vi "PicoScope5000aSetupStreaming.vi"(0 "error in":errorcluster, 1 "Device Info":T2, 2 "handle in":i16, 3 "Acquisition Settings":T3={"Auto Stop"=FALSE, "Desired Sample Interval"=4, "Pre-trigger Samples"=0, "Post-trigger Samples"=1000, "Down-Sample Ratio"=1, "Down-Sample Mode"=0, "Time Units"=2} {"Time Units" items=["Nanoseconds (ns)"=2, "Microseconds (us)"=3, "Milliseconds (ms)"=4, "Seconds (s)"=5]; "Down-Sample Mode" items=["None"=0, "Aggregate"=1, "Decimate"=2, "Average"=4]}, 4 "Buffer and Transfer Settings":T1={"startIndex"=0, "Samples"=1000000, "Down Sample Ratio"=1, "Down-Sample Mode"=0} {"Down-Sample Mode" items=["None"=0, "Aggregate"=1, "Decimate"=2, "Average"=4]; "Down Sample Ratio" step=1; "Samples" format="%_6p"}, 5 "enabled array":i16[](array[numeric]), 10 "Pointers In":u64[][](array[numeric])) -> (11 "Pointer array":u64[][](array[numeric]), 14 "error out":errorcluster, 16 "handle out":i16, 17 "Sample Interval":u32, 19 "sampleIntervalTimeUnits":u32)   [LabVIEW 2016]
doc: "Set up the data buffers and calls RunStreaming to start the device streaming.\nData will be copied from the driver buffers into the corresponding application buffers using the wrapper dll."
uses:
  ps5000a.dll
  ps5000aWrap.dll
panel:
  # "Overview Buffer Size is the size of the temporary buffers used to\nstore data before returning it to the application."
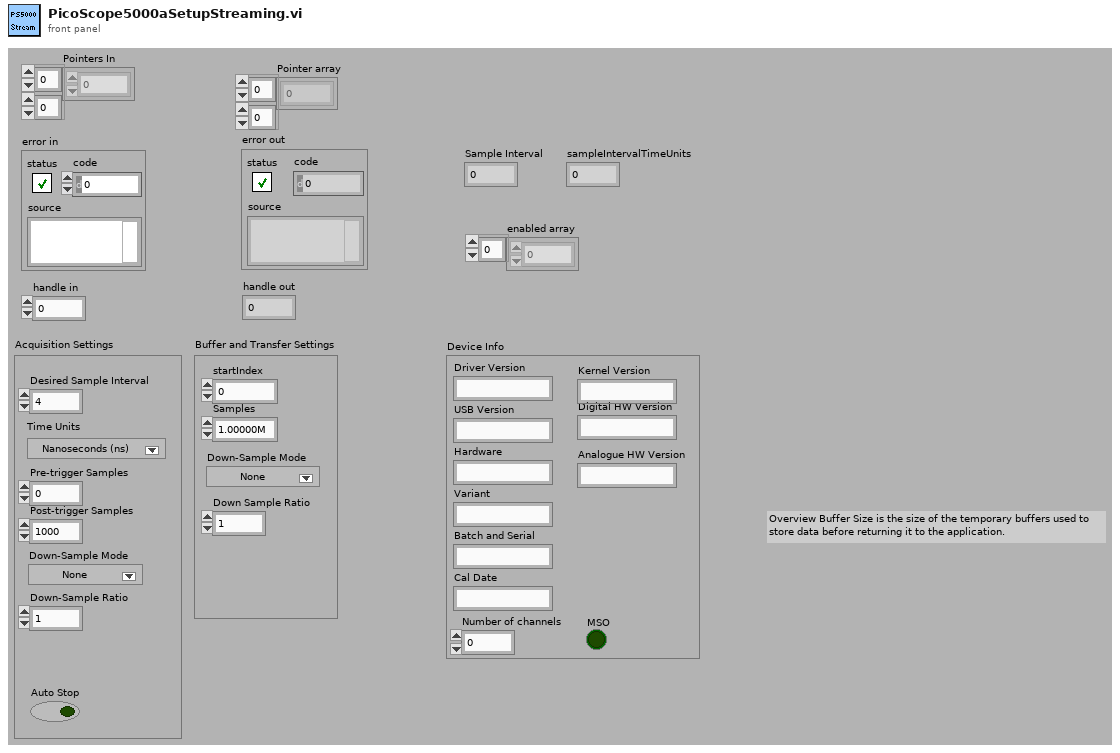
[diagram p1: front panel]
types:
  T1 = cluster{"startIndex":u64, "Samples":u64, "Down Sample Ratio":u64, "Down-Sample Mode":u32}
  T2 = cluster{"Driver Version":string, "USB Version":string, "Hardware":string, "Variant":string, "Batch and Serial":string, "Cal Date":string, "Kernel Version":string, "Digital HW Version":string, "Analogue HW Version":string, "MSO":bool, "Number of channels":i16}
  T3 = cluster{"Auto Stop":bool, "Desired Sample Interval":u32, "Pre-trigger Samples":u32, "Post-trigger Samples":u32, "Down-Sample Ratio":u32, "Down-Sample Mode":i32, "Time Units":u32}
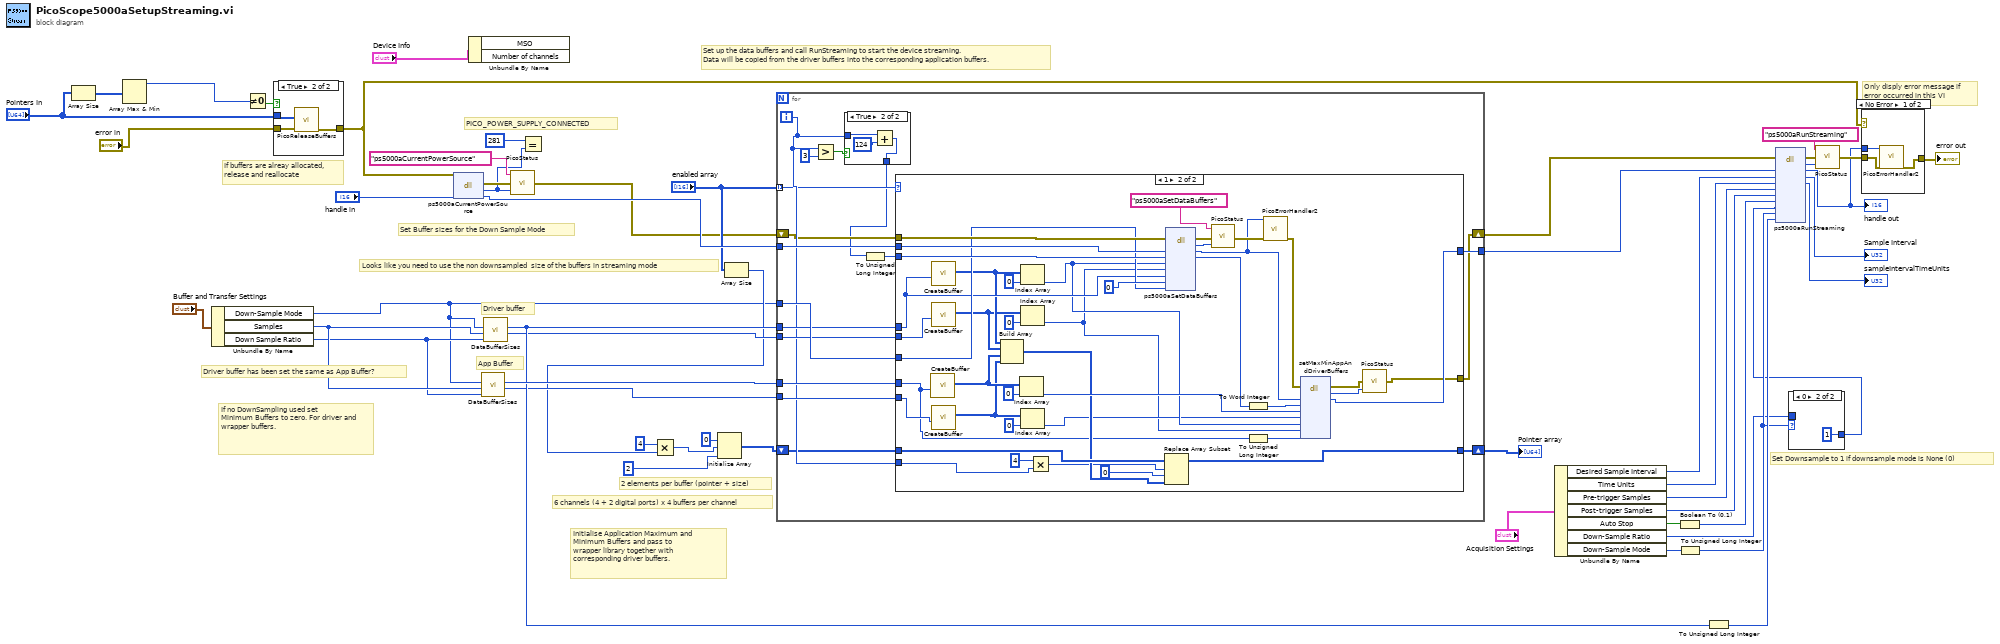
[diagram p0: block diagram]
diagram:
  # "Set Downsample to 1 if downsample mode is None (0)"
  # "Looks like you need to use the non downsampled  size of the buffers in streaming mode"
  # "If buffers are alreay allocated,\nrelease and reallocate"
  # "2 elements per buffer (pointer + size)"
  # "6 channels (4 + 2 digital ports) x 4 buffers per channel"
  # "App Buffer"
  # "Driver buffer"
  # "Driver buffer has been set the same as App Buffer?"
  # "Set Buffer sizes for the Down Sample Mode"
  # "If no DownSampling used set \nMinimum Buffers to zero. For driver and wrapper buffers."
  # "PICO_POWER_SUPPLY_CONNECTED"
  # "Initialise Application Maximum and\nMinimum Buffers and pass to \nwrapper library together with corresponding driver buffers."
  # "Only disply error message if\nerror occurred in this VI"
  # "Set up the data buffers and call RunStreaming to start the device streaming.\nData will be copied from the driver buffers into the corresponding application buffers."
  n1 = Array Size(array="Pointers In") -> (size(s)=w7:i32[])
  n2 = Array Max & Min(array=w7) -> (max value=w6:i32)  [unwired: 3 out]
  n3 = Unbundle By Name("Buffer and Transfer Settings") -> ("Down-Sample Mode"=w4:u32, "Samples"=w30:u64, "Down Sample Ratio"=w29:u64)
  n4 = Not Equal To 0?(x=w6) -> (x != 0?=w14:bool)
  n5 = case shown="True" w14 {
    tunnel: "Pointers In" -> [_ w54]
    tunnel: "error in" -> [w53 w55]
    tunnel: [w53 w56] -> w11
    frame False {
    }
    frame True {
      n6 = call "PicoReleaseBuffers.vi"("error in (no error)"=w55, "Pointer array"=w54) -> ("error out"=w56:errorcluster)  [unwired: 9 in]
    }
  }
  n7 = dll-call lib="ps5000a.dll" fn="ps5000aCurrentPowerSource"(error in=w11, "handle"="handle in") -> (error out=w37:errorcluster, "PICO_STATUS"=w35:u32, "handle"=w33:i16)  [unwired: 2 in, 1 out]
  n8 = Unbundle By Name("Device Info") -> ()  [unwired: 2 out]
  n9 = call "DataBufferSizes.vi"("Down Sample Ratio"=w29, "Number of Samples"=w30, "Down-Sample Mode"=w4) -> ("min Buffer Size"=w25:i32, "Max Buffer Size"=w28:i32)  [unwired: 7 in]
  n10 = call "DataBufferSizes.vi"("Down Sample Ratio"=w29, "Number of Samples"=w30, "Down-Sample Mode"=w4) -> ("min Buffer Size"=w26:i32, "Max Buffer Size"=w27:i32)  [unwired: 7 in]
  n11 = call "PicoStatus.vi"("PICO STATUS"=w35, "error in"=w37, "source"="ps5000aCurrentPowerSource") -> ("error out"=w10:errorcluster)
  n12 = Equal?(x=u32 281, y=w35) -> ()  [unwired: 1 out]
  n13 = Array Size(array="enabled array") -> (size(s)=w18:i32)
  n14 = Multiply(x=4, y=w18) -> (x*y=w19:i32)
  n15 = Initialize Array(u64 0 ("element"), w19, 2 ("dimension size")) -> (w8:u64[][])
  n16 = for {
    tunnel: "enabled array" -> [w62] mode=indexing
    tunnel: w33 -> [w73]
    tunnel: w4 -> [w72]
    tunnel: w28 -> [w71]
    tunnel: w27 -> [w70]
    tunnel: w26 -> [w69]
    tunnel: w25 -> [w68]
    tunnel: [w63] -> w21
    shift-right: [w61] -> w15
    shift-left: w10 -> [w60]
    shift-right: [w67] -> w24
    shift-left: w8 -> [w59]
    i -> [w64]
    n17 = Greater?(x=w64, y=3) -> (0:w65:bool)
    n18 = case shown="True" w65 {
      tunnel: [w74 w75] -> w57
      tunnel: w64 -> [w74 w77]
      frame False {
      }
      frame True {
        n19 = Add(x=w77, y=124) -> (x+y=w75:i32)
      }
    }
    n20 = To Unsigned Long Integer(number=w57) -> (unsigned 32bit integer=w58:u32)
    n21 = case shown="1" w62 {
      tunnel: w73 -> [w79 w121]
      tunnel: w60 -> [w78 w120]
      tunnel: w58 -> [_ w113]
      tunnel: w71 -> [_ w83]
      tunnel: w70 -> [_ w103]
      tunnel: w69 -> [_ w106]
      tunnel: w68 -> [_ w105]
      tunnel: w72 -> [_ w104]
      tunnel: w59 -> [w80 w97]
      tunnel: [w80 w96] -> w67
      tunnel: w64 -> [_ w93]
      tunnel: [w79 w89] -> w63
      tunnel: [w78 w88] -> w61
      frame 0, Default {
      }
      frame 1 {
        n22 = call "CreateBuffer.vi"("Buffer size"=w83) -> ("Pointer and BufferSize"=w99:u64[])  [unwired: 9 in, 1 out]
        n23 = call "CreateBuffer.vi"("Buffer size"=w103) -> ("Pointer and BufferSize"=w101:u64[])  [unwired: 9 in, 1 out]
        n24 = call "CreateBuffer.vi"("Buffer size"=w106) -> ("Pointer and BufferSize"=w100:u64[])  [unwired: 9 in, 1 out]
        n25 = call "CreateBuffer.vi"("Buffer size"=w105) -> ("Pointer and BufferSize"=w98:u64[])  [unwired: 9 in, 1 out]
        n26 = Build Array(w101, w100, w99, w98) -> (w92:u64[][])
        n27 = Index Array(array=w99, index=0) -> (element=w102:u64)
        n28 = Index Array(array=w101, index=0) -> (element=w95:u64)
        n29 = Index Array(array=w100, index=0) -> (element=w81:u64)
        n30 = Index Array(array=w98, index=0) -> (element=w82:u64)
        n31 = Multiply(x=4, y=w93) -> (x*y=w91:i32)
        n32 = Replace Array Subset(array=w97, new element=w92, index (row)=w91, index (col)=0 ("disabled index (row)")) -> (w96:u64[][])
        n33 = dll-call lib="ps5000a.dll" fn="ps5000aSetDataBuffers" ("ps3000.dll:_ps3000_open_unit@0")(error in=w120, "handle"=w121, "channel"=w113, "bufferMax"=w95, "bufferMin"=w81, "bufferLth"=w103, "segmentIndex"=u32 0, "downSampleRatioMode"=w104) -> (error out=w118:errorcluster, "PICO_STATUS"=w119:u32, "handle"=w85:i16, "channel"=w114:u32)  [unwired: 7 in, 1 out]
        n34 = call "PicoStatus.vi"("PICO STATUS"=w119, "error in"=w118, "source"="ps5000aSetDataBuffers") -> ("error out"=w87:errorcluster)
        n35 = To Word Integer(number=w114) -> (16bit integer=w115:i16)
        n36 = To Unsigned Long Integer(number=w83) -> (unsigned 32bit integer=w84:u32)
        n37 = call "PicoErrorHandler2.vi"("error in (no error)"=w87, "handle In"=w85) -> ("error out"=w86:errorcluster)  [unwired: 9 in]
        n38 = dll-call lib="ps5000aWrap.dll" fn="setMaxMinAppAndDriverBuffers"(error in=w86, "handle"=w85, "channel"=w115, "appMaxBuffer"=w102, "appMinBuffer"=w82, "driverMaxBuffer"=w95, "driverMinBuffer"=w81, "bufferLength"=w84) -> (error out=w112:errorcluster, "status"=w111:i16, "handle"=w89:i16)  [unwired: 8 in, 1 out]
        n39 = call "PicoStatus.vi"("PICO STATUS"=w111, "error in"=w112) -> ("error out"=w88:errorcluster)  [unwired: 1 in]
      }
    }
  }
  "Pointer array" <- w24
  n40 = Unbundle By Name("Acquisition Settings") -> ("Desired Sample Interval"=w45:u32, "Time Units"=w39:u32, "Pre-trigger Samples"=w44:u32, "Post-trigger Samples"=w43:u32, "Auto Stop"=w42:bool, "Down-Sample Ratio"=w2:u32, "Down-Sample Mode"=w40:i32)
  n41 = Boolean To (0,1)(Boolean=w42) -> (0, 1=w46:i16)
  n42 = To Unsigned Long Integer(number=w40) -> (unsigned 32bit integer=w3:u32)
  n43 = To Unsigned Long Integer(number=w27) -> (unsigned 32bit integer=w5:u32)
  n44 = case shown="0" w3 {
    tunnel: [w122 u32 1 ("Down-Sample Ratio")] -> w1
    tunnel: w2 -> [w122 _]
    frame Default {
    }
    frame 0 {
    }
  }
  n45 = dll-call lib="ps5000a.dll" fn="ps5000aRunStreaming" ("ps5000a.dll:_ps3000_open_unit@0")(error in=w15, "handle"=w21, "sampleInterval"=w45, "sampleIntervalTimeUnits"=w39, "maxPreTriggerSamples"=w44, "maxPostTriggerSamples"=w43, "autoStop"=w46, "downSampleRatio"=w1, "downSampleRatioMode"=w3, "overviewBufferSize"=w5) -> (error out=w50:errorcluster, "PICO_STATUS"=w51:u32, "handle"=w9:i16, "sampleInterval"=→"Sample Interval":u32, "sampleIntervalTimeUnits"=→"sampleIntervalTimeUnits":u32)  [unwired: 8 in, 1 out]
  "handle out" <- w9
  n46 = call "PicoStatus.vi"("PICO STATUS"=w51, "error in"=w50, "source"="ps5000aRunStreaming") -> ("error out"=w48:errorcluster)
  n47 = case shown="No Error" w11 {
    tunnel: [w125 w127] -> w52
    tunnel: w48 -> [w126 w127]
    tunnel: w9 -> [w124 _]
    frame No Error {
      n48 = call "PicoErrorHandler2.vi"("error in (no error)"=w126, "handle In"=w124) -> ("error out"=w125:errorcluster)  [unwired: 9 in]
    }
    frame Error {
    }
  }
  "error out" <- w52
